vi "GetLoopConditional.vi"(6 "error in":errorcluster, 9 "Loop in":refnum<class "Loop.lvclass">) -> (0 "error out":errorcluster, 3 "Loop out":refnum<class "Loop.lvclass">, 4 "conditional UID":i32)   [LabVIEW 2014, in "Loop.lvclass"]
uses:
  Loop.lvclass
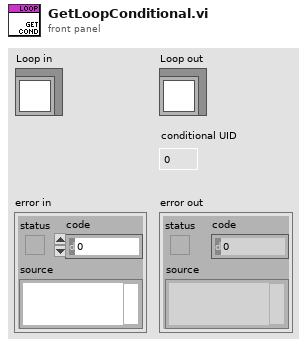
[diagram p1: front panel]
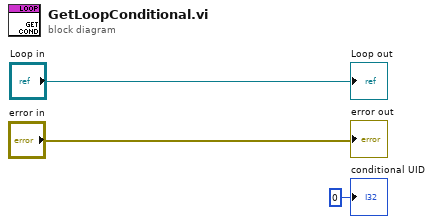
[diagram p0: block diagram]
diagram:
  "error out" <- "error in"
  "Loop out" <- "Loop in"
  "conditional UID" <- 0 ("conditional UID")
